vi "メイン.vi"() -> (2 "測定周期/ms":dbl, 3 "値転記用配列":T2[](array[typedef]))   [LabVIEW 2021] (continued)
                      n5185 = global write "測定値MAXMIN_G.vi" "測定値MAX/MINグローバル"(w7612) -> ()
                    }
                  }
                }
                frame 10 {
                  n5186 = local read "測定新値\nリセット用 11"() -> (w7613:bool)
                  n5187 = local read "測定旧値 11"() -> (w7614:bool)
                  n5188 = case shown="TRUE" w7613 {
                    frame False {
                    }
                    frame True {
                      n5189 = property on="MAX/MINグローバルリセット用" class="Arr (指定)"() -> ("Value"=w7615:string[][])  [unwired: 2 in, 2 out]
                      n5190 = global write "測定値MAXMIN_G.vi" "測定値MAX/MINグローバル"(w7615) -> ()
                    }
                  }
                  n5191 = case shown="TRUE" w7614 {
                    frame False {
                    }
                    frame True {
                      n5192 = property on="MAX/MINグローバルリセット用" class="Arr (指定)"() -> ("Value"=w7616:string[][])  [unwired: 2 in, 2 out]
                      n5193 = global write "測定値MAXMIN_G.vi" "測定値MAX/MINグローバル"(w7616) -> ()
                    }
                  }
                }
                frame 11 {
                  n5194 = local read "測定新値\nリセット用 12"() -> (w7617:bool)
                  n5195 = local read "測定旧値 12"() -> (w7618:bool)
                  n5196 = case shown="TRUE" w7617 {
                    frame False {
                    }
                    frame True {
                      n5197 = property on="MAX/MINグローバルリセット用" class="Arr (指定)"() -> ("Value"=w7619:string[][])  [unwired: 2 in, 2 out]
                      n5198 = global write "測定値MAXMIN_G.vi" "測定値MAX/MINグローバル"(w7619) -> ()
                    }
                  }
                  n5199 = case shown="TRUE" w7618 {
                    frame False {
                    }
                    frame True {
                      n5200 = property on="MAX/MINグローバルリセット用" class="Arr (指定)"() -> ("Value"=w7620:string[][])  [unwired: 2 in, 2 out]
                      n5201 = global write "測定値MAXMIN_G.vi" "測定値MAX/MINグローバル"(w7620) -> ()
                    }
                  }
                }
              }
            }
          }
          frame #1 {
            w7621 = FALSE
            # "②測定新規リセット用、測定旧値のリセット"
            n5202 = for {
              N: w7622 -> [_]
              tunnel: w7621 -> [w7626]
              i -> [w7627]
              n5203 = case shown="11" w7627 {
                tunnel: w7626 -> [w7628 w7629 w7630 w7631 w7632 w7633 w7634 w7635 w7636 w7637 w7638 w7639]
                frame 0, Default {
                  n5204 = local write "測定新値\nリセット用 1"(w7628) -> ()
                  n5205 = local write "測定旧値 1"(w7628) -> ()
                }
                frame 1 {
                  n5206 = local write "測定新値\nリセット用 2"(w7629) -> ()
                  n5207 = local write "測定旧値 2"(w7629) -> ()
                }
                frame 2 {
                  n5208 = local write "測定新値\nリセット用 3"(w7630) -> ()
                  n5209 = local write "測定旧値 3"(w7630) -> ()
                }
                frame 3 {
                  n5210 = local write "測定新値\nリセット用 4"(w7631) -> ()
                  n5211 = local write "測定旧値 4"(w7631) -> ()
                }
                frame 4 {
                  n5212 = local write "測定新値\nリセット用 5"(w7632) -> ()
                  n5213 = local write "測定旧値 5"(w7632) -> ()
                }
                frame 5 {
                  n5214 = local write "測定新値\nリセット用 6"(w7633) -> ()
                  n5215 = local write "測定旧値 6"(w7633) -> ()
                }
                frame 6 {
                  n5216 = local write "測定新値\nリセット用 7"(w7634) -> ()
                  n5217 = local write "測定旧値 7"(w7634) -> ()
                }
                frame 7 {
                  n5218 = local write "測定新値\nリセット用 8"(w7635) -> ()
                  n5219 = local write "測定旧値 8"(w7635) -> ()
                }
                frame 8 {
                  n5220 = local write "測定新値\nリセット用 9"(w7636) -> ()
                  n5221 = local write "測定旧値 9"(w7636) -> ()
                }
                frame 9 {
                  n5222 = local write "測定新値\nリセット用 10"(w7637) -> ()
                  n5223 = local write "測定旧値 10"(w7637) -> ()
                }
                frame 10 {
                  n5224 = local write "測定新値\nリセット用 11"(w7638) -> ()
                  n5225 = local write "測定旧値 11"(w7638) -> ()
                }
                frame 11 {
                  n5226 = local write "測定新値\nリセット用 12"(w7639) -> ()
                  n5227 = local write "測定旧値 12"(w7639) -> ()
                }
              }
            }
            n5228 = global write "測定キャンセルボタン.vi" "グローバル_測定キャンセルボタン"(w7621) -> ()
            n5229 = local write "G_メイン測定キャンセルボタン"(w7621) -> ()
          }
          frame #2 {
            # "⑦キュー"
            # "④グローバル_測定キャンセルボタンを\n対象測定新値がFalseならTrueにする"
            n5230 = case shown="TRUE" w7642 {
              tunnel: [_ w7652] -> w7646
              tunnel: w7645 -> [_ w7651]
              tunnel: [_ w7650] -> w7644
              tunnel: w7643 -> [_ w7649]
              tunnel: [w7647 w7648] -> w7641
              tunnel: [w7647 w7648] -> w7640
              frame False {
                w7647 = TRUE
              }
              frame True {
                w7648 = TRUE
                n5231 = Enqueue Element(queue=w7651, element="測定4", error in (no error)=w7649) -> (queue out=w7652:refnum<queue>, error out=w7650:errorcluster)  [unwired: 1 in, 1 out]
              }
            }
            n5232 = local write "G_メイン測定キャンセルボタン"(w7641) -> ()
            n5233 = global write "測定キャンセルボタン.vi" "グローバル_測定キャンセルボタン"(w7640) -> ()
          }
        }
        n5234 = for {
          N: 12 -> [_]
          tunnel: w7544 -> [w7558]
          i -> [w7559]
          n5235 = case shown="11" w7559 {
            tunnel: w7558 -> [w7560 w7561 w7562 w7563 w7564 w7565 w7566 w7567 w7568 w7569 w7570 w7571]
            frame 0, Default {
              n5236 = property on="メイン測定ボタン_単発 1" class="Bool (指定)"("DisabledEnum"=w7560) -> ()  [unwired: 2 in, 2 out]
              n5237 = property on="メイン測定ボタン_連続 1" class="Bool (指定)"("DisabledEnum"=w7560) -> ()  [unwired: 2 in, 2 out]
            }
            frame 1 {
              n5238 = property on="メイン測定ボタン_単発 2" class="Bool (指定)"("DisabledEnum"=w7561) -> ()  [unwired: 2 in, 2 out]
              n5239 = property on="メイン測定ボタン_連続 2" class="Bool (指定)"("DisabledEnum"=w7561) -> ()  [unwired: 2 in, 2 out]
            }
            frame 2 {
              n5240 = property on="メイン測定ボタン_単発 3" class="Bool (指定)"("DisabledEnum"=w7562) -> ()  [unwired: 2 in, 2 out]
              n5241 = property on="メイン測定ボタン_連続 3" class="Bool (指定)"("DisabledEnum"=w7562) -> ()  [unwired: 2 in, 2 out]
            }
            frame 3 {
              n5242 = property on="メイン測定ボタン_単発 4" class="Bool (指定)"("DisabledEnum"=w7563) -> ()  [unwired: 2 in, 2 out]
              n5243 = property on="メイン測定ボタン_連続 4" class="Bool (指定)"("DisabledEnum"=w7563) -> ()  [unwired: 2 in, 2 out]
            }
            frame 4 {
              n5244 = property on="メイン測定ボタン_単発 5" class="Bool (指定)"("DisabledEnum"=w7564) -> ()  [unwired: 2 in, 2 out]
              n5245 = property on="メイン測定ボタン_連続 5" class="Bool (指定)"("DisabledEnum"=w7564) -> ()  [unwired: 2 in, 2 out]
            }
            frame 5 {
              n5246 = property on="メイン測定ボタン_連続 6" class="Bool (指定)"("DisabledEnum"=w7565) -> ()  [unwired: 2 in, 2 out]
              n5247 = property on="メイン測定ボタン_単発 6" class="Bool (指定)"("DisabledEnum"=w7565) -> ()  [unwired: 2 in, 2 out]
            }
            frame 6 {
              n5248 = property on="メイン測定ボタン_連続 7" class="Bool (指定)"("DisabledEnum"=w7566) -> ()  [unwired: 2 in, 2 out]
              n5249 = property on="メイン測定ボタン_単発 7" class="Bool (指定)"("DisabledEnum"=w7566) -> ()  [unwired: 2 in, 2 out]
            }
            frame 7 {
              n5250 = property on="メイン測定ボタン_単発 8" class="Bool (指定)"("DisabledEnum"=w7567) -> ()  [unwired: 2 in, 2 out]
              n5251 = property on="メイン測定ボタン_連続 8" class="Bool (指定)"("DisabledEnum"=w7567) -> ()  [unwired: 2 in, 2 out]
            }
            frame 8 {
              n5252 = property on="メイン測定ボタン_単発 9" class="Bool (指定)"("DisabledEnum"=w7568) -> ()  [unwired: 2 in, 2 out]
              n5253 = property on="メイン測定ボタン_連続 9" class="Bool (指定)"("DisabledEnum"=w7568) -> ()  [unwired: 2 in, 2 out]
            }
            frame 9 {
              n5254 = property on="メイン測定ボタン_単発 10" class="Bool (指定)"("DisabledEnum"=w7569) -> ()  [unwired: 2 in, 2 out]
              n5255 = property on="メイン測定ボタン_連続 10" class="Bool (指定)"("DisabledEnum"=w7569) -> ()  [unwired: 2 in, 2 out]
            }
            frame 10 {
              n5256 = property on="メイン測定ボタン_単発 11" class="Bool (指定)"("DisabledEnum"=w7570) -> ()  [unwired: 2 in, 2 out]
              n5257 = property on="メイン測定ボタン_連続 11" class="Bool (指定)"("DisabledEnum"=w7570) -> ()  [unwired: 2 in, 2 out]
            }
            frame 11 {
              n5258 = property on="メイン測定ボタン_連続 12" class="Bool (指定)"("DisabledEnum"=w7571) -> ()  [unwired: 2 in, 2 out]
              n5259 = property on="メイン測定ボタン_単発 12" class="Bool (指定)"("DisabledEnum"=w7571) -> ()  [unwired: 2 in, 2 out]
            }
          }
        }
        n5260 = property on="TOPページへ" class="Bool"("DisabledEnum"=w7544) -> ()  [unwired: 2 in, 2 out]
        n5261 = property on="保存して終了" class="Bool"("DisabledEnum"=w7544) -> ()  [unwired: 2 in, 2 out]
        n5262 = property on="保存せずに" class="Bool"("DisabledEnum"=w7544) -> ()  [unwired: 2 in, 2 out]
      }
      event Value Change {
        w7655 = T8."Disabled" ("無効")
        # "⑤"
        # "※複製時\n①このボタンで操作する以外の\n測定旧値\n測定新値\nを複製して作る\n②ある分だけの\n測定旧値\nを複製して作る\n③ある分だけの\n測定旧値\nを複製して作る\n④はそのまま\n⑤測定新値の\nボタンが複製されているか確認\n⑥Ⅰ.初期設定の\n測定新値_リセットの初期化\nを必ず作る事\n⑦キュー"
        n5263 = event-data() -> ("NewVal"=w7664:T7)  [unwired: 1 in, 2 out]
        "測定新値 5" <- w7664
        n5264 = local read "書込周期/ms"() -> (w7654:dbl)
        n5265 = Wait (ms)(milliseconds to wait=w7654) -> ()  [unwired: 1 out]
        n5266 = flat-sequence {
          tunnel: w7664 -> [w7684]
          tunnel: w7665 -> [w7685]
          tunnel: w7667 -> [w7686]
          tunnel: [w7686] -> w7660
          tunnel: [w7685] -> w7659
          tunnel: [w7684] -> w7658
          tunnel: [w7683] -> w7657
          tunnel: [w7736] -> w7663
          tunnel: [w7735] -> w7662
          tunnel: [w7734] -> w7661
          tunnel: w7657 -> [w7732]
          tunnel: w7658 -> [w7734]
          tunnel: w7659 -> [w7735]
          tunnel: w7660 -> [w7736]
          tunnel: [w7757] -> w7668
          tunnel: [w7755] -> w7666
          tunnel: w7663 -> [w7756]
          tunnel: w7662 -> [w7754]
          tunnel: w7661 -> [w7753]
          frame #0 {
            w7683 = 32
            # "測定旧値・新値～32までTrueだったらMAX/MINグローバルリセット"
            # "①"
            n5267 = for {
              N: w7683 -> [_]
              i -> [w7687]
              n5268 = case shown="11" w7687 {
                frame 0, Default {
                  n5269 = local read "測定新値\nリセット用 1"() -> (w7688:bool)
                  n5270 = local read "測定旧値 1"() -> (w7689:bool)
                  n5271 = case shown="TRUE" w7688 {
                    frame False {
                    }
                    frame True {
                      n5272 = property on="MAX/MINグローバルリセット用" class="Arr (指定)"() -> ("Value"=w7690:string[][])  [unwired: 2 in, 2 out]
                      n5273 = global write "測定値MAXMIN_G.vi" "測定値MAX/MINグローバル"(w7690) -> ()
                    }
                  }
                  n5274 = case shown="TRUE" w7689 {
                    frame False {
                    }
                    frame True {
                      n5275 = property on="MAX/MINグローバルリセット用" class="Arr (指定)"() -> ("Value"=w7691:string[][])  [unwired: 2 in, 2 out]
                      n5276 = global write "測定値MAXMIN_G.vi" "測定値MAX/MINグローバル"(w7691) -> ()
                    }
                  }
                }
                frame 1 {
                  n5277 = local read "測定新値\nリセット用 2"() -> (w7692:bool)
                  n5278 = local read "測定旧値 2"() -> (w7693:bool)
                  n5279 = case shown="TRUE" w7692 {
                    frame False {
                    }
                    frame True {
                      n5280 = property on="MAX/MINグローバルリセット用" class="Arr (指定)"() -> ("Value"=w7694:string[][])  [unwired: 2 in, 2 out]
                      n5281 = global write "測定値MAXMIN_G.vi" "測定値MAX/MINグローバル"(w7694) -> ()
                    }
                  }
                  n5282 = case shown="TRUE" w7693 {
                    frame False {
                    }
                    frame True {
                      n5283 = property on="MAX/MINグローバルリセット用" class="Arr (指定)"() -> ("Value"=w7695:string[][])  [unwired: 2 in, 2 out]
                      n5284 = global write "測定値MAXMIN_G.vi" "測定値MAX/MINグローバル"(w7695) -> ()
                    }
                  }
                }
                frame 2 {
                  n5285 = local read "測定新値\nリセット用 3"() -> (w7696:bool)
                  n5286 = local read "測定旧値 3"() -> (w7697:bool)
                  n5287 = case shown="TRUE" w7696 {
                    frame False {
                    }
                    frame True {
                      n5288 = property on="MAX/MINグローバルリセット用" class="Arr (指定)"() -> ("Value"=w7698:string[][])  [unwired: 2 in, 2 out]
                      n5289 = global write "測定値MAXMIN_G.vi" "測定値MAX/MINグローバル"(w7698) -> ()
                    }
                  }
                  n5290 = case shown="TRUE" w7697 {
                    frame False {
                    }
                    frame True {
                      n5291 = property on="MAX/MINグローバルリセット用" class="Arr (指定)"() -> ("Value"=w7699:string[][])  [unwired: 2 in, 2 out]
                      n5292 = global write "測定値MAXMIN_G.vi" "測定値MAX/MINグローバル"(w7699) -> ()
                    }
                  }
                }
                frame 3 {
                  n5293 = local read "測定新値\nリセット用 4"() -> (w7700:bool)
                  n5294 = local read "測定旧値 4"() -> (w7701:bool)
                  n5295 = case shown="TRUE" w7700 {
                    frame False {
                    }
                    frame True {
                      n5296 = property on="MAX/MINグローバルリセット用" class="Arr (指定)"() -> ("Value"=w7702:string[][])  [unwired: 2 in, 2 out]
                      n5297 = global write "測定値MAXMIN_G.vi" "測定値MAX/MINグローバル"(w7702) -> ()
                    }
                  }
                  n5298 = case shown="TRUE" w7701 {
                    frame False {
                    }
                    frame True {
                      n5299 = property on="MAX/MINグローバルリセット用" class="Arr (指定)"() -> ("Value"=w7703:string[][])  [unwired: 2 in, 2 out]
                      n5300 = global write "測定値MAXMIN_G.vi" "測定値MAX/MINグローバル"(w7703) -> ()
                    }
                  }
                }
                frame 5 {
                  n5301 = local read "測定旧値 6"() -> (w7704:bool)
                  n5302 = local read "測定旧値 6"() -> (w7705:bool)
                  n5303 = case shown="TRUE" w7704 {
                    frame False {
                    }
                    frame True {
                      n5304 = property on="MAX/MINグローバルリセット用" class="Arr (指定)"() -> ("Value"=w7706:string[][])  [unwired: 2 in, 2 out]
                      n5305 = global write "測定値MAXMIN_G.vi" "測定値MAX/MINグローバル"(w7706) -> ()
                    }
                  }
                  n5306 = case shown="TRUE" w7705 {
                    frame False {
                    }
                    frame True {
                      n5307 = property on="MAX/MINグローバルリセット用" class="Arr (指定)"() -> ("Value"=w7707:string[][])  [unwired: 2 in, 2 out]
                      n5308 = global write "測定値MAXMIN_G.vi" "測定値MAX/MINグローバル"(w7707) -> ()
                    }
                  }
                }
                frame 6 {
                  n5309 = local read "測定旧値 7"() -> (w7708:bool)
                  n5310 = local read "測定旧値 7"() -> (w7709:bool)
                  n5311 = case shown="TRUE" w7708 {
                    frame False {
                    }
                    frame True {
                      n5312 = property on="MAX/MINグローバルリセット用" class="Arr (指定)"() -> ("Value"=w7710:string[][])  [unwired: 2 in, 2 out]
                      n5313 = global write "測定値MAXMIN_G.vi" "測定値MAX/MINグローバル"(w7710) -> ()
                    }
                  }
                  n5314 = case shown="TRUE" w7709 {
                    frame False {
                    }
                    frame True {
                      n5315 = property on="MAX/MINグローバルリセット用" class="Arr (指定)"() -> ("Value"=w7711:string[][])  [unwired: 2 in, 2 out]
                      n5316 = global write "測定値MAXMIN_G.vi" "測定値MAX/MINグローバル"(w7711) -> ()
                    }
                  }
                }
                frame 7 {
                  n5317 = local read "測定新値\nリセット用 8"() -> (w7712:bool)
                  n5318 = local read "測定旧値 8"() -> (w7713:bool)
                  n5319 = case shown="TRUE" w7712 {
                    frame False {
                    }
                    frame True {
                      n5320 = property on="MAX/MINグローバルリセット用" class="Arr (指定)"() -> ("Value"=w7714:string[][])  [unwired: 2 in, 2 out]
                      n5321 = global write "測定値MAXMIN_G.vi" "測定値MAX/MINグローバル"(w7714) -> ()
                    }
                  }
                  n5322 = case shown="TRUE" w7713 {
                    frame False {
                    }
                    frame True {
                      n5323 = property on="MAX/MINグローバルリセット用" class="Arr (指定)"() -> ("Value"=w7715:string[][])  [unwired: 2 in, 2 out]
                      n5324 = global write "測定値MAXMIN_G.vi" "測定値MAX/MINグローバル"(w7715) -> ()
                    }
                  }
                }
                frame 8 {
                  n5325 = local read "測定新値\nリセット用 9"() -> (w7716:bool)
                  n5326 = local read "測定旧値 9"() -> (w7717:bool)
                  n5327 = case shown="TRUE" w7716 {
                    frame False {
                    }
                    frame True {
                      n5328 = property on="MAX/MINグローバルリセット用" class="Arr (指定)"() -> ("Value"=w7718:string[][])  [unwired: 2 in, 2 out]
                      n5329 = global write "測定値MAXMIN_G.vi" "測定値MAX/MINグローバル"(w7718) -> ()
                    }
                  }
                  n5330 = case shown="TRUE" w7717 {
                    frame False {
                    }
                    frame True {
                      n5331 = property on="MAX/MINグローバルリセット用" class="Arr (指定)"() -> ("Value"=w7719:string[][])  [unwired: 2 in, 2 out]
                      n5332 = global write "測定値MAXMIN_G.vi" "測定値MAX/MINグローバル"(w7719) -> ()
                    }
                  }
                }
                frame 9 {
                  n5333 = local read "測定新値\nリセット用 10"() -> (w7720:bool)
                  n5334 = local read "測定旧値 10"() -> (w7721:bool)
                  n5335 = case shown="TRUE" w7720 {
                    frame False {
                    }
                    frame True {
                      n5336 = property on="MAX/MINグローバルリセット用" class="Arr (指定)"() -> ("Value"=w7722:string[][])  [unwired: 2 in, 2 out]
                      n5337 = global write "測定値MAXMIN_G.vi" "測定値MAX/MINグローバル"(w7722) -> ()
                    }
                  }
                  n5338 = case shown="TRUE" w7721 {
                    frame False {
                    }
                    frame True {
                      n5339 = property on="MAX/MINグローバルリセット用" class="Arr (指定)"() -> ("Value"=w7723:string[][])  [unwired: 2 in, 2 out]
                      n5340 = global write "測定値MAXMIN_G.vi" "測定値MAX/MINグローバル"(w7723) -> ()
                    }
                  }
                }
                frame 10 {
                  n5341 = local read "測定新値\nリセット用 11"() -> (w7724:bool)
                  n5342 = local read "測定旧値 11"() -> (w7725:bool)
                  n5343 = case shown="TRUE" w7724 {
                    frame False {
                    }
                    frame True {
                      n5344 = property on="MAX/MINグローバルリセット用" class="Arr (指定)"() -> ("Value"=w7726:string[][])  [unwired: 2 in, 2 out]
                      n5345 = global write "測定値MAXMIN_G.vi" "測定値MAX/MINグローバル"(w7726) -> ()
                    }
                  }
                  n5346 = case shown="TRUE" w7725 {
                    frame False {
                    }
                    frame True {
                      n5347 = property on="MAX/MINグローバルリセット用" class="Arr (指定)"() -> ("Value"=w7727:string[][])  [unwired: 2 in, 2 out]
                      n5348 = global write "測定値MAXMIN_G.vi" "測定値MAX/MINグローバル"(w7727) -> ()
                    }
                  }
                }
                frame 11 {
                  n5349 = local read "測定新値\nリセット用 12"() -> (w7728:bool)
                  n5350 = local read "測定旧値 12"() -> (w7729:bool)
                  n5351 = case shown="TRUE" w7728 {
                    frame False {
                    }
                    frame True {
                      n5352 = property on="MAX/MINグローバルリセット用" class="Arr (指定)"() -> ("Value"=w7730:string[][])  [unwired: 2 in, 2 out]
                      n5353 = global write "測定値MAXMIN_G.vi" "測定値MAX/MINグローバル"(w7730) -> ()
                    }
                  }
                  n5354 = case shown="TRUE" w7729 {
                    frame False {
                    }
                    frame True {
                      n5355 = property on="MAX/MINグローバルリセット用" class="Arr (指定)"() -> ("Value"=w7731:string[][])  [unwired: 2 in, 2 out]
                      n5356 = global write "測定値MAXMIN_G.vi" "測定値MAX/MINグローバル"(w7731) -> ()
                    }
                  }
                }
              }
            }
          }
          frame #1 {
            w7733 = FALSE
            # "②測定新規リセット用、測定旧値のリセット"
            n5357 = for {
              N: w7732 -> [_]
              tunnel: w7733 -> [w7737]
              i -> [w7738]
              n5358 = case shown="11" w7738 {
                tunnel: w7737 -> [w7739 w7740 w7741 w7742 w7743 w7744 w7745 w7746 w7747 w7748 w7749 w7750]
                frame 0, Default {
                  n5359 = local write "測定新値\nリセット用 1"(w7739) -> ()
                  n5360 = local write "測定旧値 1"(w7739) -> ()
                }
                frame 1 {
                  n5361 = local write "測定新値\nリセット用 2"(w7740) -> ()
                  n5362 = local write "測定旧値 2"(w7740) -> ()
                }
                frame 2 {
                  n5363 = local write "測定新値\nリセット用 3"(w7741) -> ()
                  n5364 = local write "測定旧値 3"(w7741) -> ()
                }
                frame 3 {
                  n5365 = local write "測定新値\nリセット用 4"(w7742) -> ()
                  n5366 = local write "測定旧値 4"(w7742) -> ()
                }
                frame 4 {
                  n5367 = local write "測定新値\nリセット用 5"(w7743) -> ()
                  n5368 = local write "測定旧値 5"(w7743) -> ()
                }
                frame 5 {
                  n5369 = local write "測定新値\nリセット用 6"(w7744) -> ()
                  n5370 = local write "測定旧値 6"(w7744) -> ()
                }
                frame 6 {
                  n5371 = local write "測定新値\nリセット用 7"(w7745) -> ()
                  n5372 = local write "測定旧値 7"(w7745) -> ()
                }
                frame 7 {
                  n5373 = local write "測定新値\nリセット用 8"(w7746) -> ()
                  n5374 = local write "測定旧値 8"(w7746) -> ()
                }
                frame 8 {
                  n5375 = local write "測定新値\nリセット用 9"(w7747) -> ()
                  n5376 = local write "測定旧値 9"(w7747) -> ()
                }
                frame 9 {
                  n5377 = local write "測定新値\nリセット用 10"(w7748) -> ()
                  n5378 = local write "測定旧値 10"(w7748) -> ()
                }
                frame 10 {
                  n5379 = local write "測定新値\nリセット用 11"(w7749) -> ()
                  n5380 = local write "測定旧値 11"(w7749) -> ()
                }
                frame 11 {
                  n5381 = local write "測定新値\nリセット用 12"(w7750) -> ()
                  n5382 = local write "測定旧値 12"(w7750) -> ()
                }
              }
            }
            n5383 = global write "測定キャンセルボタン.vi" "グローバル_測定キャンセルボタン"(w7733) -> ()
            n5384 = local write "G_メイン測定キャンセルボタン"(w7733) -> ()
          }
          frame #2 {
            # "⑦キュー"
            # "④グローバル_測定キャンセルボタンを\n対象測定新値がFalseならTrueにする"
            n5385 = case shown="TRUE" w7753 {
              tunnel: [_ w7763] -> w7757
              tunnel: w7756 -> [_ w7762]
              tunnel: [_ w7761] -> w7755
              tunnel: w7754 -> [_ w7760]
              tunnel: [w7758 w7759] -> w7752
              tunnel: [w7758 w7759] -> w7751
              frame False {
                w7758 = TRUE
              }
              frame True {
                w7759 = TRUE
                n5386 = Enqueue Element(queue=w7762, element="測定5", error in (no error)=w7760) -> (queue out=w7763:refnum<queue>, error out=w7761:errorcluster)  [unwired: 1 in, 1 out]
              }
            }
            n5387 = local write "G_メイン測定キャンセルボタン"(w7752) -> ()
            n5388 = global write "測定キャンセルボタン.vi" "グローバル_測定キャンセルボタン"(w7751) -> ()
          }
        }
        n5389 = for {
          N: 12 -> [_]
          tunnel: w7655 -> [w7669]
          i -> [w7670]
          n5390 = case shown="11" w7670 {
            tunnel: w7669 -> [w7671 w7672 w7673 w7674 w7675 w7676 w7677 w7678 w7679 w7680 w7681 w7682]
            frame 0, Default {
              n5391 = property on="メイン測定ボタン_単発 1" class="Bool (指定)"("DisabledEnum"=w7671) -> ()  [unwired: 2 in, 2 out]
              n5392 = property on="メイン測定ボタン_連続 1" class="Bool (指定)"("DisabledEnum"=w7671) -> ()  [unwired: 2 in, 2 out]
            }
            frame 1 {
              n5393 = property on="メイン測定ボタン_単発 2" class="Bool (指定)"("DisabledEnum"=w7672) -> ()  [unwired: 2 in, 2 out]
              n5394 = property on="メイン測定ボタン_連続 2" class="Bool (指定)"("DisabledEnum"=w7672) -> ()  [unwired: 2 in, 2 out]
            }
            frame 2 {
              n5395 = property on="メイン測定ボタン_単発 3" class="Bool (指定)"("DisabledEnum"=w7673) -> ()  [unwired: 2 in, 2 out]
              n5396 = property on="メイン測定ボタン_連続 3" class="Bool (指定)"("DisabledEnum"=w7673) -> ()  [unwired: 2 in, 2 out]
            }
            frame 3 {
              n5397 = property on="メイン測定ボタン_単発 4" class="Bool (指定)"("DisabledEnum"=w7674) -> ()  [unwired: 2 in, 2 out]
              n5398 = property on="メイン測定ボタン_連続 4" class="Bool (指定)"("DisabledEnum"=w7674) -> ()  [unwired: 2 in, 2 out]
            }
            frame 4 {
              n5399 = property on="メイン測定ボタン_単発 5" class="Bool (指定)"("DisabledEnum"=w7675) -> ()  [unwired: 2 in, 2 out]
              n5400 = property on="メイン測定ボタン_連続 5" class="Bool (指定)"("DisabledEnum"=w7675) -> ()  [unwired: 2 in, 2 out]
            }
            frame 5 {
              n5401 = property on="メイン測定ボタン_連続 6" class="Bool (指定)"("DisabledEnum"=w7676) -> ()  [unwired: 2 in, 2 out]
              n5402 = property on="メイン測定ボタン_単発 6" class="Bool (指定)"("DisabledEnum"=w7676) -> ()  [unwired: 2 in, 2 out]
            }
            frame 6 {
              n5403 = property on="メイン測定ボタン_連続 7" class="Bool (指定)"("DisabledEnum"=w7677) -> ()  [unwired: 2 in, 2 out]
              n5404 = property on="メイン測定ボタン_単発 7" class="Bool (指定)"("DisabledEnum"=w7677) -> ()  [unwired: 2 in, 2 out]
            }
            frame 7 {
              n5405 = property on="メイン測定ボタン_単発 8" class="Bool (指定)"("DisabledEnum"=w7678) -> ()  [unwired: 2 in, 2 out]
              n5406 = property on="メイン測定ボタン_連続 8" class="Bool (指定)"("DisabledEnum"=w7678) -> ()  [unwired: 2 in, 2 out]
            }
            frame 8 {
              n5407 = property on="メイン測定ボタン_単発 9" class="Bool (指定)"("DisabledEnum"=w7679) -> ()  [unwired: 2 in, 2 out]
              n5408 = property on="メイン測定ボタン_連続 9" class="Bool (指定)"("DisabledEnum"=w7679) -> ()  [unwired: 2 in, 2 out]
            }
            frame 9 {
              n5409 = property on="メイン測定ボタン_単発 10" class="Bool (指定)"("DisabledEnum"=w7680) -> ()  [unwired: 2 in, 2 out]
              n5410 = property on="メイン測定ボタン_連続 10" class="Bool (指定)"("DisabledEnum"=w7680) -> ()  [unwired: 2 in, 2 out]
            }
            frame 10 {
              n5411 = property on="メイン測定ボタン_単発 11" class="Bool (指定)"("DisabledEnum"=w7681) -> ()  [unwired: 2 in, 2 out]
              n5412 = property on="メイン測定ボタン_連続 11" class="Bool (指定)"("DisabledEnum"=w7681) -> ()  [unwired: 2 in, 2 out]
            }
            frame 11 {
              n5413 = property on="メイン測定ボタン_連続 12" class="Bool (指定)"("DisabledEnum"=w7682) -> ()  [unwired: 2 in, 2 out]
              n5414 = property on="メイン測定ボタン_単発 12" class="Bool (指定)"("DisabledEnum"=w7682) -> ()  [unwired: 2 in, 2 out]
            }
          }
        }
        n5415 = property on="TOPページへ" class="Bool"("DisabledEnum"=w7655) -> ()  [unwired: 2 in, 2 out]
        n5416 = property on="保存して終了" class="Bool"("DisabledEnum"=w7655) -> ()  [unwired: 2 in, 2 out]
        n5417 = property on="保存せずに" class="Bool"("DisabledEnum"=w7655) -> ()  [unwired: 2 in, 2 out]
      }
      event Value Change {
        w7766 = T8."Disabled" ("無効")
        # "⑤"
        # "※複製時\n①このボタンで操作する以外の\n測定旧値\n測定新値\nを複製して作る\n②ある分だけの\n測定旧値\nを複製して作る\n③ある分だけの\n測定旧値\nを複製して作る\n④はそのまま\n⑤測定新値の\nボタンが複製されているか確認\n⑥Ⅰ.初期設定の\n測定新値_リセットの初期化\nを必ず作る事\n⑦キュー"
        n5418 = event-data() -> ("NewVal"=w7775:T7)  [unwired: 1 in, 2 out]
        "測定新値 6" <- w7775
        n5419 = local read "書込周期/ms"() -> (w7765:dbl)
        n5420 = Wait (ms)(milliseconds to wait=w7765) -> ()  [unwired: 1 out]
        n5421 = flat-sequence {
          tunnel: w7775 -> [w7795]
          tunnel: w7776 -> [w7796]
          tunnel: w7778 -> [w7797]
          tunnel: [w7797] -> w7771
          tunnel: [w7796] -> w7770
          tunnel: [w7795] -> w7769
          tunnel: [w7794] -> w7768
          tunnel: [w7847] -> w7774
          tunnel: [w7846] -> w7773
          tunnel: [w7845] -> w7772
          tunnel: w7768 -> [w7844]
          tunnel: w7769 -> [w7845]
          tunnel: w7770 -> [w7846]
          tunnel: w7771 -> [w7847]
          tunnel: [w7868] -> w7779
          tunnel: [w7866] -> w7777
          tunnel: w7774 -> [w7867]
          tunnel: w7773 -> [w7865]
          tunnel: w7772 -> [w7864]
          frame #0 {
            w7794 = 32
            # "測定旧値・新値～32までTrueだったらMAX/MINグローバルリセット"
            # "①"
            n5422 = for {
              N: w7794 -> [_]
              i -> [w7798]
              n5423 = case shown="11" w7798 {
                frame 0, Default {
                  n5424 = local read "測定新値\nリセット用 1"() -> (w7799:bool)
                  n5425 = local read "測定旧値 1"() -> (w7800:bool)
                  n5426 = case shown="TRUE" w7799 {
                    frame False {
                    }
                    frame True {
                      n5427 = property on="MAX/MINグローバルリセット用" class="Arr (指定)"() -> ("Value"=w7801:string[][])  [unwired: 2 in, 2 out]
                      n5428 = global write "測定値MAXMIN_G.vi" "測定値MAX/MINグローバル"(w7801) -> ()
                    }
                  }
                  n5429 = case shown="TRUE" w7800 {
                    frame False {
                    }
                    frame True {
                      n5430 = property on="MAX/MINグローバルリセット用" class="Arr (指定)"() -> ("Value"=w7802:string[][])  [unwired: 2 in, 2 out]
                      n5431 = global write "測定値MAXMIN_G.vi" "測定値MAX/MINグローバル"(w7802) -> ()
                    }
                  }
                }
                frame 1 {
                  n5432 = local read "測定新値\nリセット用 2"() -> (w7803:bool)
                  n5433 = local read "測定旧値 2"() -> (w7804:bool)
                  n5434 = case shown="TRUE" w7803 {
                    frame False {
                    }
                    frame True {
                      n5435 = property on="MAX/MINグローバルリセット用" class="Arr (指定)"() -> ("Value"=w7805:string[][])  [unwired: 2 in, 2 out]
                      n5436 = global write "測定値MAXMIN_G.vi" "測定値MAX/MINグローバル"(w7805) -> ()
                    }
                  }
                  n5437 = case shown="TRUE" w7804 {
                    frame False {
                    }
                    frame True {
                      n5438 = property on="MAX/MINグローバルリセット用" class="Arr (指定)"() -> ("Value"=w7806:string[][])  [unwired: 2 in, 2 out]
                      n5439 = global write "測定値MAXMIN_G.vi" "測定値MAX/MINグローバル"(w7806) -> ()
                    }
                  }
                }
                frame 2 {
                  n5440 = local read "測定新値\nリセット用 3"() -> (w7807:bool)
                  n5441 = local read "測定旧値 3"() -> (w7808:bool)
                  n5442 = case shown="TRUE" w7807 {
                    frame False {
                    }
                    frame True {
                      n5443 = property on="MAX/MINグローバルリセット用" class="Arr (指定)"() -> ("Value"=w7809:string[][])  [unwired: 2 in, 2 out]
                      n5444 = global write "測定値MAXMIN_G.vi" "測定値MAX/MINグローバル"(w7809) -> ()
                    }
                  }
                  n5445 = case shown="TRUE" w7808 {
                    frame False {
                    }
                    frame True {
                      n5446 = property on="MAX/MINグローバルリセット用" class="Arr (指定)"() -> ("Value"=w7810:string[][])  [unwired: 2 in, 2 out]
                      n5447 = global write "測定値MAXMIN_G.vi" "測定値MAX/MINグローバル"(w7810) -> ()
                    }
                  }
                }
                frame 3 {
                  n5448 = local read "測定新値\nリセット用 4"() -> (w7811:bool)
                  n5449 = local read "測定旧値 4"() -> (w7812:bool)
                  n5450 = case shown="TRUE" w7811 {
                    frame False {
                    }
                    frame True {
                      n5451 = property on="MAX/MINグローバルリセット用" class="Arr (指定)"() -> ("Value"=w7813:string[][])  [unwired: 2 in, 2 out]
                      n5452 = global write "測定値MAXMIN_G.vi" "測定値MAX/MINグローバル"(w7813) -> ()
                    }
                  }
                  n5453 = case shown="TRUE" w7812 {
                    frame False {
                    }
                    frame True {
                      n5454 = property on="MAX/MINグローバルリセット用" class="Arr (指定)"() -> ("Value"=w7814:string[][])  [unwired: 2 in, 2 out]
                      n5455 = global write "測定値MAXMIN_G.vi" "測定値MAX/MINグローバル"(w7814) -> ()
                    }
                  }
                }
                frame 4 {
                  n5456 = local read "測定新値\nリセット用 5"() -> (w7815:bool)
                  n5457 = local read "測定旧値 5"() -> (w7816:bool)
                  n5458 = case shown="TRUE" w7815 {
                    frame False {
                    }
                    frame True {
                      n5459 = property on="MAX/MINグローバルリセット用" class="Arr (指定)"() -> ("Value"=w7817:string[][])  [unwired: 2 in, 2 out]
                      n5460 = global write "測定値MAXMIN_G.vi" "測定値MAX/MINグローバル"(w7817) -> ()
                    }
                  }
                  n5461 = case shown="TRUE" w7816 {
                    frame False {
                    }
                    frame True {
                      n5462 = property on="MAX/MINグローバルリセット用" class="Arr (指定)"() -> ("Value"=w7818:string[][])  [unwired: 2 in, 2 out]
                      n5463 = global write "測定値MAXMIN_G.vi" "測定値MAX/MINグローバル"(w7818) -> ()
                    }
                  }
                }
                frame 6 {
                  n5464 = local read "測定新値\nリセット用 7"() -> (w7819:bool)
                  n5465 = local read "測定旧値 7"() -> (w7820:bool)
                  n5466 = case shown="TRUE" w7819 {
                    frame False {
                    }
                    frame True {
                      n5467 = property on="MAX/MINグローバルリセット用" class="Arr (指定)"() -> ("Value"=w7821:string[][])  [unwired: 2 in, 2 out]
                      n5468 = global write "測定値MAXMIN_G.vi" "測定値MAX/MINグローバル"(w7821) -> ()
                    }
                  }
                  n5469 = case shown="TRUE" w7820 {
                    frame False {
                    }
                    frame True {
                      n5470 = property on="MAX/MINグローバルリセット用" class="Arr (指定)"() -> ("Value"=w7822:string[][])  [unwired: 2 in, 2 out]
                      n5471 = global write "測定値MAXMIN_G.vi" "測定値MAX/MINグローバル"(w7822) -> ()
                    }
                  }
                }
                frame 7 {
                  n5472 = local read "測定新値\nリセット用 8"() -> (w7823:bool)
                  n5473 = local read "測定旧値 8"() -> (w7824:bool)
                  n5474 = case shown="TRUE" w7823 {
                    frame False {
                    }
                    frame True {
                      n5475 = property on="MAX/MINグローバルリセット用" class="Arr (指定)"() -> ("Value"=w7825:string[][])  [unwired: 2 in, 2 out]
                      n5476 = global write "測定値MAXMIN_G.vi" "測定値MAX/MINグローバル"(w7825) -> ()
                    }
                  }
                  n5477 = case shown="TRUE" w7824 {
                    frame False {
                    }
                    frame True {
                      n5478 = property on="MAX/MINグローバルリセット用" class="Arr (指定)"() -> ("Value"=w7826:string[][])  [unwired: 2 in, 2 out]
                      n5479 = global write "測定値MAXMIN_G.vi" "測定値MAX/MINグローバル"(w7826) -> ()
                    }
                  }
                }
                frame 8 {
                  n5480 = local read "測定新値\nリセット用 9"() -> (w7827:bool)
                  n5481 = local read "測定旧値 9"() -> (w7828:bool)
                  n5482 = case shown="TRUE" w7827 {
                    frame False {
                    }
                    frame True {
                      n5483 = property on="MAX/MINグローバルリセット用" class="Arr (指定)"() -> ("Value"=w7829:string[][])  [unwired: 2 in, 2 out]
                      n5484 = global write "測定値MAXMIN_G.vi" "測定値MAX/MINグローバル"(w7829) -> ()
                    }
                  }
                  n5485 = case shown="TRUE" w7828 {
                    frame False {
                    }
                    frame True {
                      n5486 = property on="MAX/MINグローバルリセット用" class="Arr (指定)"() -> ("Value"=w7830:string[][])  [unwired: 2 in, 2 out]
                      n5487 = global write "測定値MAXMIN_G.vi" "測定値MAX/MINグローバル"(w7830) -> ()
                    }
                  }
                }
                frame 9 {
                  n5488 = local read "測定新値\nリセット用 10"() -> (w7831:bool)
                  n5489 = local read "測定旧値 10"() -> (w7832:bool)
                  n5490 = case shown="TRUE" w7831 {
                    frame False {
                    }
                    frame True {
                      n5491 = property on="MAX/MINグローバルリセット用" class="Arr (指定)"() -> ("Value"=w7833:string[][])  [unwired: 2 in, 2 out]
                      n5492 = global write "測定値MAXMIN_G.vi" "測定値MAX/MINグローバル"(w7833) -> ()
                    }
                  }
                  n5493 = case shown="TRUE" w7832 {
                    frame False {
                    }
                    frame True {
                      n5494 = property on="MAX/MINグローバルリセット用" class="Arr (指定)"() -> ("Value"=w7834:string[][])  [unwired: 2 in, 2 out]
                      n5495 = global write "測定値MAXMIN_G.vi" "測定値MAX/MINグローバル"(w7834) -> ()
                    }
                  }
                }
                frame 10 {
                  n5496 = local read "測定新値\nリセット用 11"() -> (w7835:bool)
                  n5497 = local read "測定旧値 11"() -> (w7836:bool)
                  n5498 = case shown="TRUE" w7835 {
                    frame False {
                    }
                    frame True {
                      n5499 = property on="MAX/MINグローバルリセット用" class="Arr (指定)"() -> ("Value"=w7837:string[][])  [unwired: 2 in, 2 out]
                      n5500 = global write "測定値MAXMIN_G.vi" "測定値MAX/MINグローバル"(w7837) -> ()
                    }
                  }
                  n5501 = case shown="TRUE" w7836 {
                    frame False {
                    }
                    frame True {
                      n5502 = property on="MAX/MINグローバルリセット用" class="Arr (指定)"() -> ("Value"=w7838:string[][])  [unwired: 2 in, 2 out]
                      n5503 = global write "測定値MAXMIN_G.vi" "測定値MAX/MINグローバル"(w7838) -> ()
                    }
                  }
                }
                frame 11 {
                  n5504 = local read "測定新値\nリセット用 12"() -> (w7839:bool)
                  n5505 = local read "測定旧値 12"() -> (w7840:bool)
                  n5506 = case shown="TRUE" w7839 {
                    frame False {
                    }
                    frame True {
                      n5507 = property on="MAX/MINグローバルリセット用" class="Arr (指定)"() -> ("Value"=w7841:string[][])  [unwired: 2 in, 2 out]
                      n5508 = global write "測定値MAXMIN_G.vi" "測定値MAX/MINグローバル"(w7841) -> ()
                    }
                  }
                  n5509 = case shown="TRUE" w7840 {
                    frame False {
                    }
                    frame True {
                      n5510 = property on="MAX/MINグローバルリセット用" class="Arr (指定)"() -> ("Value"=w7842:string[][])  [unwired: 2 in, 2 out]
                      n5511 = global write "測定値MAXMIN_G.vi" "測定値MAX/MINグローバル"(w7842) -> ()
                    }
                  }
                }
              }
            }
          }
          frame #1 {
            w7843 = FALSE
            # "②測定新規リセット用、測定旧値のリセット"
            n5512 = for {
              N: w7844 -> [_]
              tunnel: w7843 -> [w7848]
              i -> [w7849]
              n5513 = case shown="11" w7849 {
                tunnel: w7848 -> [w7850 w7851 w7852 w7853 w7854 w7855 w7856 w7857 w7858 w7859 w7860 w7861]
                frame 0, Default {
                  n5514 = local write "測定新値\nリセット用 1"(w7850) -> ()
                  n5515 = local write "測定旧値 1"(w7850) -> ()
                }
                frame 1 {
                  n5516 = local write "測定新値\nリセット用 2"(w7851) -> ()
                  n5517 = local write "測定旧値 2"(w7851) -> ()
                }
                frame 2 {
                  n5518 = local write "測定新値\nリセット用 3"(w7852) -> ()
                  n5519 = local write "測定旧値 3"(w7852) -> ()
                }
                frame 3 {
                  n5520 = local write "測定新値\nリセット用 4"(w7853) -> ()
                  n5521 = local write "測定旧値 4"(w7853) -> ()
                }
                frame 4 {
                  n5522 = local write "測定新値\nリセット用 5"(w7854) -> ()
                  n5523 = local write "測定旧値 5"(w7854) -> ()
                }
                frame 5 {
                  n5524 = local write "測定新値\nリセット用 6"(w7855) -> ()
                  n5525 = local write "測定旧値 6"(w7855) -> ()
                }
                frame 6 {
                  n5526 = local write "測定新値\nリセット用 7"(w7856) -> ()
                  n5527 = local write "測定旧値 7"(w7856) -> ()
                }
                frame 7 {
                  n5528 = local write "測定新値\nリセット用 8"(w7857) -> ()
                  n5529 = local write "測定旧値 8"(w7857) -> ()
                }
                frame 8 {
                  n5530 = local write "測定新値\nリセット用 9"(w7858) -> ()
                  n5531 = local write "測定旧値 9"(w7858) -> ()
                }
                frame 9 {
                  n5532 = local write "測定新値\nリセット用 10"(w7859) -> ()
                  n5533 = local write "測定旧値 10"(w7859) -> ()
                }
                frame 10 {
                  n5534 = local write "測定新値\nリセット用 11"(w7860) -> ()
                  n5535 = local write "測定旧値 11"(w7860) -> ()
                }
                frame 11 {
                  n5536 = local write "測定新値\nリセット用 12"(w7861) -> ()
                  n5537 = local write "測定旧値 12"(w7861) -> ()
                }
              }
            }
            n5538 = global write "測定キャンセルボタン.vi" "グローバル_測定キャンセルボタン"(w7843) -> ()
            n5539 = local write "G_メイン測定キャンセルボタン"(w7843) -> ()
          }
          frame #2 {
            # "⑦キュー"
            # "④グローバル_測定キャンセルボタンを\n対象測定新値がFalseならTrueにする"
            n5540 = case shown="TRUE" w7864 {
              tunnel: [_ w7874] -> w7868
              tunnel: w7867 -> [_ w7873]
              tunnel: [_ w7872] -> w7866
              tunnel: w7865 -> [_ w7871]
              tunnel: [w7869 w7870] -> w7863
              tunnel: [w7869 w7870] -> w7862
              frame False {
                w7869 = TRUE
              }
              frame True {
                w7870 = TRUE
                n5541 = Enqueue Element(queue=w7873, element="測定6", error in (no error)=w7871) -> (queue out=w7874:refnum<queue>, error out=w7872:errorcluster)  [unwired: 1 in, 1 out]
              }
            }
            n5542 = local write "G_メイン測定キャンセルボタン"(w7863) -> ()
            n5543 = global write "測定キャンセルボタン.vi" "グローバル_測定キャンセルボタン"(w7862) -> ()
          }
        }
        n5544 = for {
          N: 12 -> [_]
          tunnel: w7766 -> [w7780]
          i -> [w7781]
          n5545 = case shown="11" w7781 {
            tunnel: w7780 -> [w7782 w7783 w7784 w7785 w7786 w7787 w7788 w7789 w7790 w7791 w7792 w7793]
            frame 0, Default {
              n5546 = property on="メイン測定ボタン_単発 1" class="Bool (指定)"("DisabledEnum"=w7782) -> ()  [unwired: 2 in, 2 out]
              n5547 = property on="メイン測定ボタン_連続 1" class="Bool (指定)"("DisabledEnum"=w7782) -> ()  [unwired: 2 in, 2 out]
            }
            frame 1 {
              n5548 = property on="メイン測定ボタン_単発 2" class="Bool (指定)"("DisabledEnum"=w7783) -> ()  [unwired: 2 in, 2 out]
              n5549 = property on="メイン測定ボタン_連続 2" class="Bool (指定)"("DisabledEnum"=w7783) -> ()  [unwired: 2 in, 2 out]
            }
            frame 2 {
              n5550 = property on="メイン測定ボタン_単発 3" class="Bool (指定)"("DisabledEnum"=w7784) -> ()  [unwired: 2 in, 2 out]
              n5551 = property on="メイン測定ボタン_連続 3" class="Bool (指定)"("DisabledEnum"=w7784) -> ()  [unwired: 2 in, 2 out]
            }
            frame 3 {
              n5552 = property on="メイン測定ボタン_単発 4" class="Bool (指定)"("DisabledEnum"=w7785) -> ()  [unwired: 2 in, 2 out]
              n5553 = property on="メイン測定ボタン_連続 4" class="Bool (指定)"("DisabledEnum"=w7785) -> ()  [unwired: 2 in, 2 out]
            }
            frame 4 {
              n5554 = property on="メイン測定ボタン_単発 5" class="Bool (指定)"("DisabledEnum"=w7786) -> ()  [unwired: 2 in, 2 out]
              n5555 = property on="メイン測定ボタン_連続 5" class="Bool (指定)"("DisabledEnum"=w7786) -> ()  [unwired: 2 in, 2 out]
            }
            frame 5 {
              n5556 = property on="メイン測定ボタン_連続 6" class="Bool (指定)"("DisabledEnum"=w7787) -> ()  [unwired: 2 in, 2 out]
              n5557 = property on="メイン測定ボタン_単発 6" class="Bool (指定)"("DisabledEnum"=w7787) -> ()  [unwired: 2 in, 2 out]
            }
            frame 6 {
              n5558 = property on="メイン測定ボタン_連続 7" class="Bool (指定)"("DisabledEnum"=w7788) -> ()  [unwired: 2 in, 2 out]
              n5559 = property on="メイン測定ボタン_単発 7" class="Bool (指定)"("DisabledEnum"=w7788) -> ()  [unwired: 2 in, 2 out]
            }
            frame 7 {
              n5560 = property on="メイン測定ボタン_単発 8" class="Bool (指定)"("DisabledEnum"=w7789) -> ()  [unwired: 2 in, 2 out]
              n5561 = property on="メイン測定ボタン_連続 8" class="Bool (指定)"("DisabledEnum"=w7789) -> ()  [unwired: 2 in, 2 out]
            }
            frame 8 {
              n5562 = property on="メイン測定ボタン_単発 9" class="Bool (指定)"("DisabledEnum"=w7790) -> ()  [unwired: 2 in, 2 out]
              n5563 = property on="メイン測定ボタン_連続 9" class="Bool (指定)"("DisabledEnum"=w7790) -> ()  [unwired: 2 in, 2 out]
            }
            frame 9 {
              n5564 = property on="メイン測定ボタン_単発 10" class="Bool (指定)"("DisabledEnum"=w7791) -> ()  [unwired: 2 in, 2 out]
              n5565 = property on="メイン測定ボタン_連続 10" class="Bool (指定)"("DisabledEnum"=w7791) -> ()  [unwired: 2 in, 2 out]
            }
            frame 10 {
              n5566 = property on="メイン測定ボタン_単発 11" class="Bool (指定)"("DisabledEnum"=w7792) -> ()  [unwired: 2 in, 2 out]
              n5567 = property on="メイン測定ボタン_連続 11" class="Bool (指定)"("DisabledEnum"=w7792) -> ()  [unwired: 2 in, 2 out]
            }
            frame 11 {
              n5568 = property on="メイン測定ボタン_連続 12" class="Bool (指定)"("DisabledEnum"=w7793) -> ()  [unwired: 2 in, 2 out]
              n5569 = property on="メイン測定ボタン_単発 12" class="Bool (指定)"("DisabledEnum"=w7793) -> ()  [unwired: 2 in, 2 out]
            }
          }
        }
        n5570 = property on="TOPページへ" class="Bool"("DisabledEnum"=w7766) -> ()  [unwired: 2 in, 2 out]
        n5571 = property on="保存して終了" class="Bool"("DisabledEnum"=w7766) -> ()  [unwired: 2 in, 2 out]
        n5572 = property on="保存せずに" class="Bool"("DisabledEnum"=w7766) -> ()  [unwired: 2 in, 2 out]
      }
      event Value Change {
        w7877 = T8."Disabled" ("無効")
        # "⑤"
        # "※複製時\n①このボタンで操作する以外の\n測定旧値\n測定新値\nを複製して作る\n②ある分だけの\n測定旧値\nを複製して作る\n③ある分だけの\n測定旧値\nを複製して作る\n④はそのまま\n⑤測定新値の\nボタンが複製されているか確認\n⑥Ⅰ.初期設定の\n測定新値_リセットの初期化\nを必ず作る事\n⑦キュー"
        n5573 = event-data() -> ("NewVal"=w7886:T7)  [unwired: 1 in, 2 out]
        "測定新値 7" <- w7886
        n5574 = local read "書込周期/ms"() -> (w7876:dbl)
        n5575 = Wait (ms)(milliseconds to wait=w7876) -> ()  [unwired: 1 out]
        n5576 = flat-sequence {
          tunnel: w7886 -> [w7906]
          tunnel: w7887 -> [w7907]
          tunnel: w7889 -> [w7908]
          tunnel: [w7908] -> w7882
          tunnel: [w7907] -> w7881
          tunnel: [w7906] -> w7880
          tunnel: [w7905] -> w7879
          tunnel: [w7958] -> w7885
          tunnel: [w7957] -> w7884
          tunnel: [w7956] -> w7883
          tunnel: w7879 -> [w7955]
          tunnel: w7880 -> [w7956]
          tunnel: w7881 -> [w7957]
          tunnel: w7882 -> [w7958]
          tunnel: [w7979] -> w7890
          tunnel: [w7977] -> w7888
          tunnel: w7885 -> [w7978]
          tunnel: w7884 -> [w7976]
          tunnel: w7883 -> [w7975]
          frame #0 {
            w7905 = 32
            # "測定旧値・新値～32までTrueだったらMAX/MINグローバルリセット"
            # "①"
            n5577 = for {
              N: w7905 -> [_]
              i -> [w7909]
              n5578 = case shown="11" w7909 {
                frame 0, Default {
                  n5579 = local read "測定新値\nリセット用 1"() -> (w7910:bool)
                  n5580 = local read "測定旧値 1"() -> (w7911:bool)
                  n5581 = case shown="TRUE" w7910 {
                    frame False {
                    }
                    frame True {
                      n5582 = property on="MAX/MINグローバルリセット用" class="Arr (指定)"() -> ("Value"=w7912:string[][])  [unwired: 2 in, 2 out]
                      n5583 = global write "測定値MAXMIN_G.vi" "測定値MAX/MINグローバル"(w7912) -> ()
                    }
                  }
                  n5584 = case shown="TRUE" w7911 {
                    frame False {
                    }
                    frame True {
                      n5585 = property on="MAX/MINグローバルリセット用" class="Arr (指定)"() -> ("Value"=w7913:string[][])  [unwired: 2 in, 2 out]
                      n5586 = global write "測定値MAXMIN_G.vi" "測定値MAX/MINグローバル"(w7913) -> ()
                    }
                  }
                }
                frame 1 {
                  n5587 = local read "測定新値\nリセット用 2"() -> (w7914:bool)
                  n5588 = local read "測定旧値 2"() -> (w7915:bool)
                  n5589 = case shown="TRUE" w7914 {
                    frame False {
                    }
                    frame True {
                      n5590 = property on="MAX/MINグローバルリセット用" class="Arr (指定)"() -> ("Value"=w7916:string[][])  [unwired: 2 in, 2 out]
                      n5591 = global write "測定値MAXMIN_G.vi" "測定値MAX/MINグローバル"(w7916) -> ()
                    }
                  }
                  n5592 = case shown="TRUE" w7915 {
                    frame False {
                    }
                    frame True {
                      n5593 = property on="MAX/MINグローバルリセット用" class="Arr (指定)"() -> ("Value"=w7917:string[][])  [unwired: 2 in, 2 out]
                      n5594 = global write "測定値MAXMIN_G.vi" "測定値MAX/MINグローバル"(w7917) -> ()
                    }
                  }
                }
                frame 2 {
                  n5595 = local read "測定新値\nリセット用 3"() -> (w7918:bool)
                  n5596 = local read "測定旧値 3"() -> (w7919:bool)
                  n5597 = case shown="TRUE" w7918 {
                    frame False {
                    }
                    frame True {
                      n5598 = property on="MAX/MINグローバルリセット用" class="Arr (指定)"() -> ("Value"=w7920:string[][])  [unwired: 2 in, 2 out]
                      n5599 = global write "測定値MAXMIN_G.vi" "測定値MAX/MINグローバル"(w7920) -> ()
                    }
                  }
                  n5600 = case shown="TRUE" w7919 {
                    frame False {
                    }
                    frame True {
                      n5601 = property on="MAX/MINグローバルリセット用" class="Arr (指定)"() -> ("Value"=w7921:string[][])  [unwired: 2 in, 2 out]
                      n5602 = global write "測定値MAXMIN_G.vi" "測定値MAX/MINグローバル"(w7921) -> ()
                    }
                  }
                }
                frame 3 {
                  n5603 = local read "測定新値\nリセット用 4"() -> (w7922:bool)
                  n5604 = local read "測定旧値 4"() -> (w7923:bool)
                  n5605 = case shown="TRUE" w7922 {
                    frame False {
                    }
                    frame True {
                      n5606 = property on="MAX/MINグローバルリセット用" class="Arr (指定)"() -> ("Value"=w7924:string[][])  [unwired: 2 in, 2 out]
                      n5607 = global write "測定値MAXMIN_G.vi" "測定値MAX/MINグローバル"(w7924) -> ()
                    }
                  }
                  n5608 = case shown="TRUE" w7923 {
                    frame False {
                    }
                    frame True {
                      n5609 = property on="MAX/MINグローバルリセット用" class="Arr (指定)"() -> ("Value"=w7925:string[][])  [unwired: 2 in, 2 out]
                      n5610 = global write "測定値MAXMIN_G.vi" "測定値MAX/MINグローバル"(w7925) -> ()
                    }
                  }
                }
                frame 4 {
                  n5611 = local read "測定新値\nリセット用 5"() -> (w7926:bool)
                  n5612 = local read "測定旧値 5"() -> (w7927:bool)
                  n5613 = case shown="TRUE" w7926 {
                    frame False {
                    }
                    frame True {
                      n5614 = property on="MAX/MINグローバルリセット用" class="Arr (指定)"() -> ("Value"=w7928:string[][])  [unwired: 2 in, 2 out]
                      n5615 = global write "測定値MAXMIN_G.vi" "測定値MAX/MINグローバル"(w7928) -> ()
                    }
                  }
                  n5616 = case shown="TRUE" w7927 {
                    frame False {
                    }
                    frame True {
                      n5617 = property on="MAX/MINグローバルリセット用" class="Arr (指定)"() -> ("Value"=w7929:string[][])  [unwired: 2 in, 2 out]
